vi "Panel Create.vi"(10 "Actor":refnum<class "Actor.lvclass">, 11 "Panel in":refnum<class "Panel.lvclass">) -> (0 "error out":errorcluster, 3 "Panel out":refnum<class "Panel.lvclass">)   [LabVIEW 2021, in "Panel.lvclass"]
uses:
  Panel.lvclass
  <vilib>/jettl/jettl/jettl/Actor/Actor.lvclass
  Panel Wrapper.vi
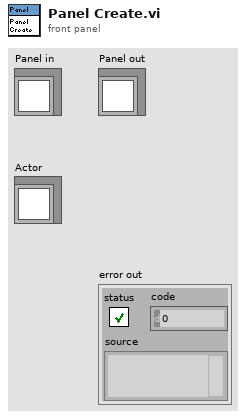
[diagram p1: front panel]
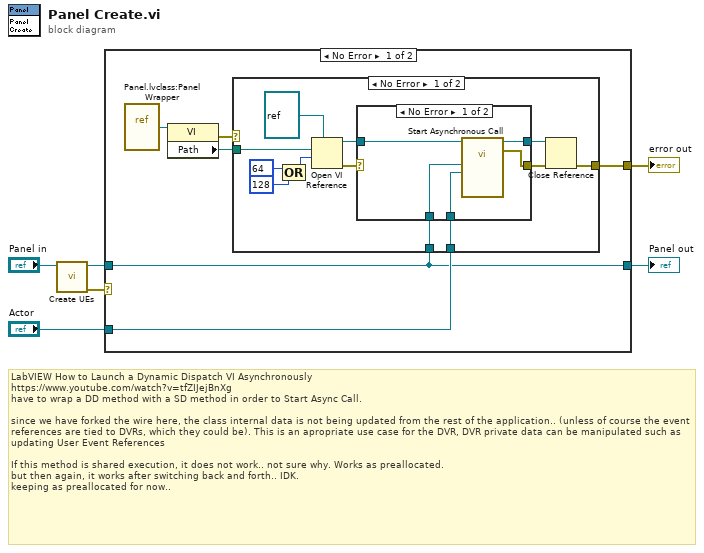
[diagram p0: block diagram]
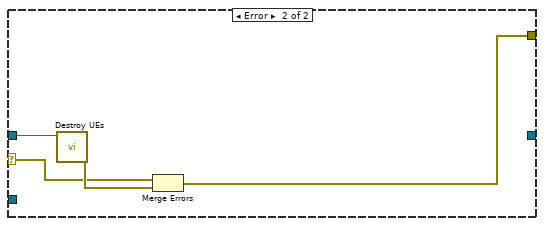
[diagram p4: hidden frame]
diagram:
  # "LabVIEW How to Launch a Dynamic Dispatch VI Asynchronously\nhttps://www.youtube.com/watch?v=tfZIJejBnXg\nhave to wrap a DD method with a SD method in order to Start Async Call.\n\nsince we have forked the wire here, the class internal data is not being updated from the rest of the application.. (unless of course the event references are tied to DVRs, which they could be). This is an apropriate use case for the DVR, DVR private data can be manipulated such as updating User Event References\n\nIf this method is shared execution, it does not work.. not sure why. Works as preallocated.\nbut then again, it works after switching back and forth.. IDK.\nkeeping as preallocated for now.."
  n1 = call-dynamic "Create UEs.vi"("Panel in"="Panel in") -> ("error out"=w3:errorcluster, "Panel out"=w2:refnum<class "Panel.lvclass">)  [unwired: 9 in]
  n2 = case shown="No Error" w3 {
    selector: w3 -> [_ w33]
    tunnel: [w12 w34] -> w6
    tunnel: "Actor" -> [w8 _]
    tunnel: w2 -> [w7 w36]
    tunnel: [w7 _] -> w1
    frame No Error {
      n3 = vi-ref "Panel.lvclass:Panel Wrapper.vi"() -> (w10:refnum<vi>)
      n4 = property class="VI"(reference=w10) -> (error out=w11:errorcluster, "Path"=w9:path)  [unwired: 1 in, 1 out]
      n5 = case shown="No Error" w11 {
        selector: w11 -> [_ w32]
        tunnel: [w22 w32] -> w12
        tunnel: w9 -> [w15 _]
        tunnel: w8 -> [w14 _]
        tunnel: w7 -> [w13 _]
        frame No Error {
          n6 = Compound Arithmetic op=OR(64 ("options: Multiple Clones,\n  Fire & Forget"), 128 ("options: Multiple Clones,\n  Fire & Forget")) -> (w20:i32)
          n7 = Open VI Reference(type specifier VI Refnum (for type only)=refnum<vi> refnum, vi path=w15, options=w20) -> (vi reference=w17:refnum<vi>, error out=w18:errorcluster)  [unwired: 3 in]
          n8 = case shown="No Error" w18 {
            selector: w18 -> [_ w31]
            tunnel: [w28 w30] -> w24
            tunnel: [w27 w31] -> w23
            tunnel: w17 -> [w29 w30]
            tunnel: w14 -> [w26 _]
            tunnel: w13 -> [w25 _]
            frame No Error {
              n9 = call-by-ref "Start Asynchronous Call"(reference=w29, "Actor"=w26, "Panel in"=w25) -> (reference out=w28:refnum<vi>, error out=w27:errorcluster)  [unwired: 11 in]
            }
            frame Error {
            }
          }
          n10 = Close Reference(reference=w24, error in (no error)=w23) -> (error out=w22:errorcluster)
        }
        frame Error {
        }
      }
    }
    frame Error {
      n11 = call-dynamic "Destroy UEs.vi"("Panel in"=w36) -> ("error out"=w35:errorcluster)  [unwired: 10 in]
      n12 = Merge Errors(w33, w35) -> (w34:errorcluster)
    }
  }
  "error out" <- w6
  "Panel out" <- w1
